vi "PH_Cont-601k_PowerUnit.write PSDB.vi"(0 "i ref in":refnum<vi>, 5 "error IO":errorcluster) -> (14 "i ref out":refnum<vi>, 19 "error out":errorcluster)   [LabVIEW 2014, in "PH_Cont-601k_PowerUnit.lvlib"]
doc: "This is the proc case which writes data to the PHELIX shot data base."
uses:
  PH_Cont-601k_PowerUnit.lvlib
  PH_Basics/PH_PowerUnit_BaseClass/PH_PowerUnit_BaseClass.SM States.ctl
  PH_Basics/PH_PSDBWriter/PH_PSDBWriter.lvlib
  PH_Basics/PH_PowerUnit_BaseClass/PH_PowerUnit_BaseClass.lvlib
  CS_Core/BaseSM/BaseSM.lvlib
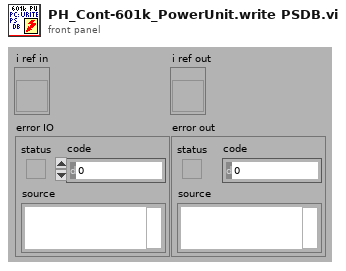
[diagram p1: front panel]
types:
  T1 = typedef "PH_PowerUnit_BaseClass.lvlib/PH_PowerUnit_BaseClass.i attribute.ctl" = cluster{"Constructor finished":bool, "PU":cluster{"In use":bool, "Service ID in use":i32, "GUI Ref":refnum<vi>}, "Enabling":cluster{"State":T2, "GUI Ref":refnum<vi>}, "Timing":cluster{"Last Shot":dbl, "Time between Shots [Sec]":dbl, "Waiting Time over?":bool, "Service ID Waiting Time":i32, "GUI Ref":refnum<vi>, "Instance":cluster{"Status":T3, "linked?":bool, "GUI Ref":refnum<vi>}}, "Sequencer":cluster{"SM State":string, "GUI Ref":refnum<vi>, "linked":bool}, "Subscribed Trendmssgs":cluster{"Tagname":string, "Status":T3, "linked?":bool, "Shot Condition":T3, "GUI Ref":refnum<vi>}[], "PP PU":T4, "Default Voltage (V)":dbl, "GUI Refs":T5, "PSDB data":cluster{"Shot Voltage [V]":dbl, "State TO SM":T6, "Write 2 early":bool}, "State TO SM":T6}
  T2 = typedef "PH_SystemInformation.lvlib/PH_SystemInformationEnabling State.ctl" = i32
  T3 = typedef "PH_StatusHandler.lvlib/PH_StatusHandler.Status.ctl" = i16
  T4 = typedef "PH_PP_Common.lvlib/PH_PP_Common.PUs.ctl" = enum16{"no Info", "PA-19mm-1", "PA-19mm-2", "PA-45mm-PILC", "PA-45mm-MAIN", "MA-PU-1", "MA-PU-2", "MA-PU-3", "MA-PU-4", "MA-PU-5", "MA-PU-6", "MA-FR", "MA-PILC", "PA-45mm-DP"}
  T5 = typedef "PH_PowerUnit_BaseClass.lvlib/PH_PowerUnit_BaseClass.GUI Refs.ctl" = cluster{"Delete Inst":refnum<vi>, "State TO SM":refnum<vi>, "State SM":refnum<vi>, "Fire":refnum<vi>}
  T6 = typedef "PH_PowerUnit_BaseClass.lvlib/PH_PowerUnit_BaseClass.SM States.ctl" = enum16{".", "Stand by", "Switch PU on", "Configure", "Set Default Voltage", "Set STANDBY", "Set READY", "Wait for Shot Cmd", "Open Dump Rods", "Open Ross Relais", "Close Ross Relais", "Switch PSU on", "Switch PSU off", "Charge", "Switch GD Channel on", "Close Dump Rods", "Rods-TO", "RR-TO", "PSU-TO", "Trigger-TO"}
  T7 = typedef "PH_PSDBWriter.lvlib/PH_PSDBWriter.Boolean dataset.ctl" = cluster{"name":string, "data":bool, "unit":string}
  T8 = typedef "PH_PSDBWriter.lvlib/PH_PSDBWriter.String dataset.ctl" = cluster{"name":string, "data":string, "unit":string}
  T9 = typedef "PH_PSDBWriter.lvlib/PH_PSDBWriter.Numeric dataset.ctl" = cluster{"name":string, "data":dbl, "unit":string}
  T10 = typedef "PH_PSDBWriter.lvlib/PH_PSDBWriter.PSDB Dataset.ctl" = cluster{"Version":i32, "2D data Input":T11[], "Boolean Input":T7[], "Image Input":T13[], "Numeric Input":T9[], "String Input":T8[]}
  T11 = typedef "PH_PSDBWriter.lvlib/PH_PSDBWriter.2D dataset.ctl" = cluster{"name":string, "data":dbl[][], "axis description":T12}
  T12 = typedef "PSDB.lvlib/PSDB_AxisDescription.ctl" = cluster{"x axis label":string, "y axis label":string, "x axis unit":string, "y axis unit":string}
  T13 = typedef "PH_PSDBWriter.lvlib/PH_PSDBWriter.Image dataset.ctl" = cluster{"name":string, "data":T14, "unit":string}
  T14 = typedef "IMAQ Image.ctl" = refnum<image>
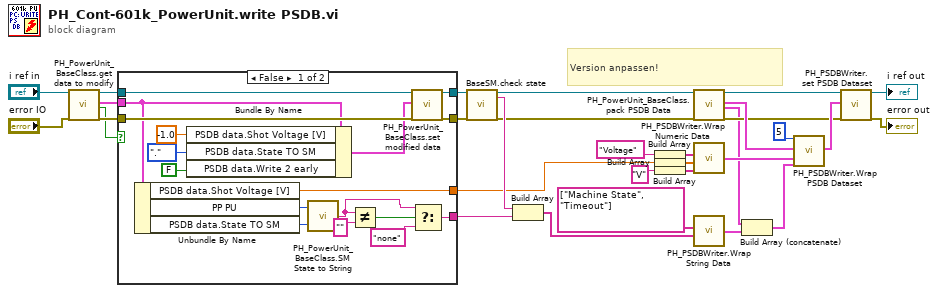
[diagram p0: block diagram]
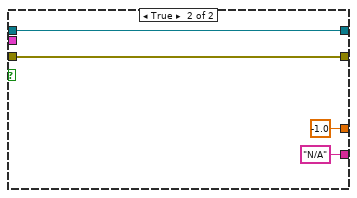
[diagram p2: hidden frame]
diagram:
  # "Version anpassen!"
  n1 = call "PH_PowerUnit_BaseClass.get data to modify.vi"("i ref in"="i ref in", "error in (no error)"="error IO") -> ("i ref out"=w18:refnum<vi>, "i attribute"=w16:T1, "timed out"=w15:bool, "error out"=w17:errorcluster)  [unwired: 14 in]
  n2 = case shown="False" w15 {
    tunnel: w18 -> [w48 w52]
    tunnel: w17 -> [w47 w51]
    tunnel: [w46 w52] -> w13
    tunnel: [w45 w51] -> w14
    tunnel: [w44 -1.0 ("Shot Voltage [V]")] -> w4
    tunnel: w16 -> [w43 _]
    tunnel: [w32 "N/A" ("State TO SM")] -> w9
    frame False {
      n3 = Unbundle By Name(w43) -> ("PSDB data.Shot Voltage [V]"=w44:dbl, "PP PU"=w37:T4, "PSDB data.State TO SM"=w40:T6)
      n4 = Bundle By Name(cluster=w43, "PSDB data.Shot Voltage [V]"=-1.0, "PSDB data.State TO SM"=PH_PowerUnit_BaseClass.SM_States.".", "PSDB data.Write 2 early"=FALSE) -> (w42:T1)
      n5 = call "PH_PowerUnit_BaseClass.SM State to String.vi"("SM State"=w40, "PU"=w37) -> ("SM State String"=w33:string)
      n6 = Not Equal?(x=w33, y="") -> (x != y?=w35:bool)
      n7 = call "PH_PowerUnit_BaseClass.set modified data.vi"("i ref in"=w48, "i attribute"=w42, "error in (no error)"=w47) -> ("i ref out"=w46:refnum<vi>, "error out"=w45:errorcluster)  [unwired: 15 in]
      n8 = Select(t=w33, s=w35, f="none") -> (s? t:f=w32:string)
    }
    frame True {
    }
  }
  n9 = call "BaseSM.check state.vi"("i ref in"=w13, "error in (no error)"=w14) -> ("i ref out"=w6:refnum<vi>, "actualState"=w10:string, "error out"=w5:errorcluster)  [unwired: 12 in, 3 out]
  n10 = Build Array(w10, w9) -> (w11:string[])
  n11 = Build Array("Voltage" ("name")) -> (w25:string[])
  n12 = Build Array(w4) -> (w26:dbl[])
  n13 = Build Array("V" ("unit")) -> (w24:string[])
  n14 = call "PH_PowerUnit_BaseClass.pack PSDB Data.vi"("VI in"=w6, "error in (no error)"=w5) -> ("VI out"=w21:refnum<vi>, "PSDB Boolean Data Array"=w20:T7[], "PSDB String Data Array"=w3:T8[], "error out"=w19:errorcluster)  [unwired: 14 in]
  n15 = call "PH_PSDBWriter.Wrap Numeric Data.vi"("Unit Array"=w24, "Data Array"=w26, "Name Array"=w25) -> ("PSDB Numeric Data Array"=w23:T9[])  [unwired: 1 in]
  n16 = call "PH_PSDBWriter.Wrap String Data.vi"("Data Array"=w11, "Name Array"=string[] ["Machine State", "Timeout"]) -> ("PSDB String Data Array"=w12:T8[])  [unwired: 2 in]
  n17 = Build Array (concatenate)(w3, w12) -> (w2:T8[])
  n18 = call "PH_PSDBWriter.Wrap PSDB Dataset.vi"("Version"=5, "Boolean Input"=w20, "Numeric Input"=w23, "String Input"=w2) -> ("PSDB Dataset"=w22:T10)  [unwired: 15 in]
  n19 = call "PH_PSDBWriter.set PSDB Dataset.vi"("VI in"=w21, "PSDB Dataset"=w22, "error in (no error)"=w19) -> ("VI out"=→"i ref out":refnum<vi>, "error out"=→"error out":errorcluster)  [unwired: 15 in]
